vi "Quaternary_Layer2.vi"(2 "Debug Mode":bool, 3 "Elapsed Time (s)":dbl, 4 "State":enum16{"Edit", "Start", "Run", "End", "Idle"}(ring), 5 "Argument List In":string[](array[string])) -> (0 "Status Out":string, 1 "Argument List Out":string[](array[string]))   [LabVIEW 2011]
panel:
  in  "PH3 run":bool
  in  "AsH3 run":bool
  in  "In run":bool
  in  "Ga run":bool
  in  "PH3 Flow":dbl
  in  "AsH3 Flow":dbl
  in  "In Flow":dbl
  in  "Ga Flow":dbl
  in  "Cancel":bool
  in  "OK":bool
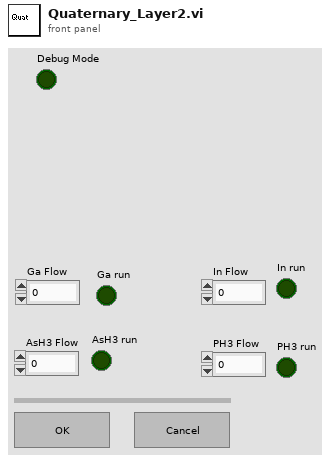
[diagram p1: front panel]
types:
  T1 = enum16{"Discrete", "Continuous", "Instantaneous"}
  T2 = enum32{"Invalid", "Default", "Floating", "Floating/Auto-Hide", "Modal"}
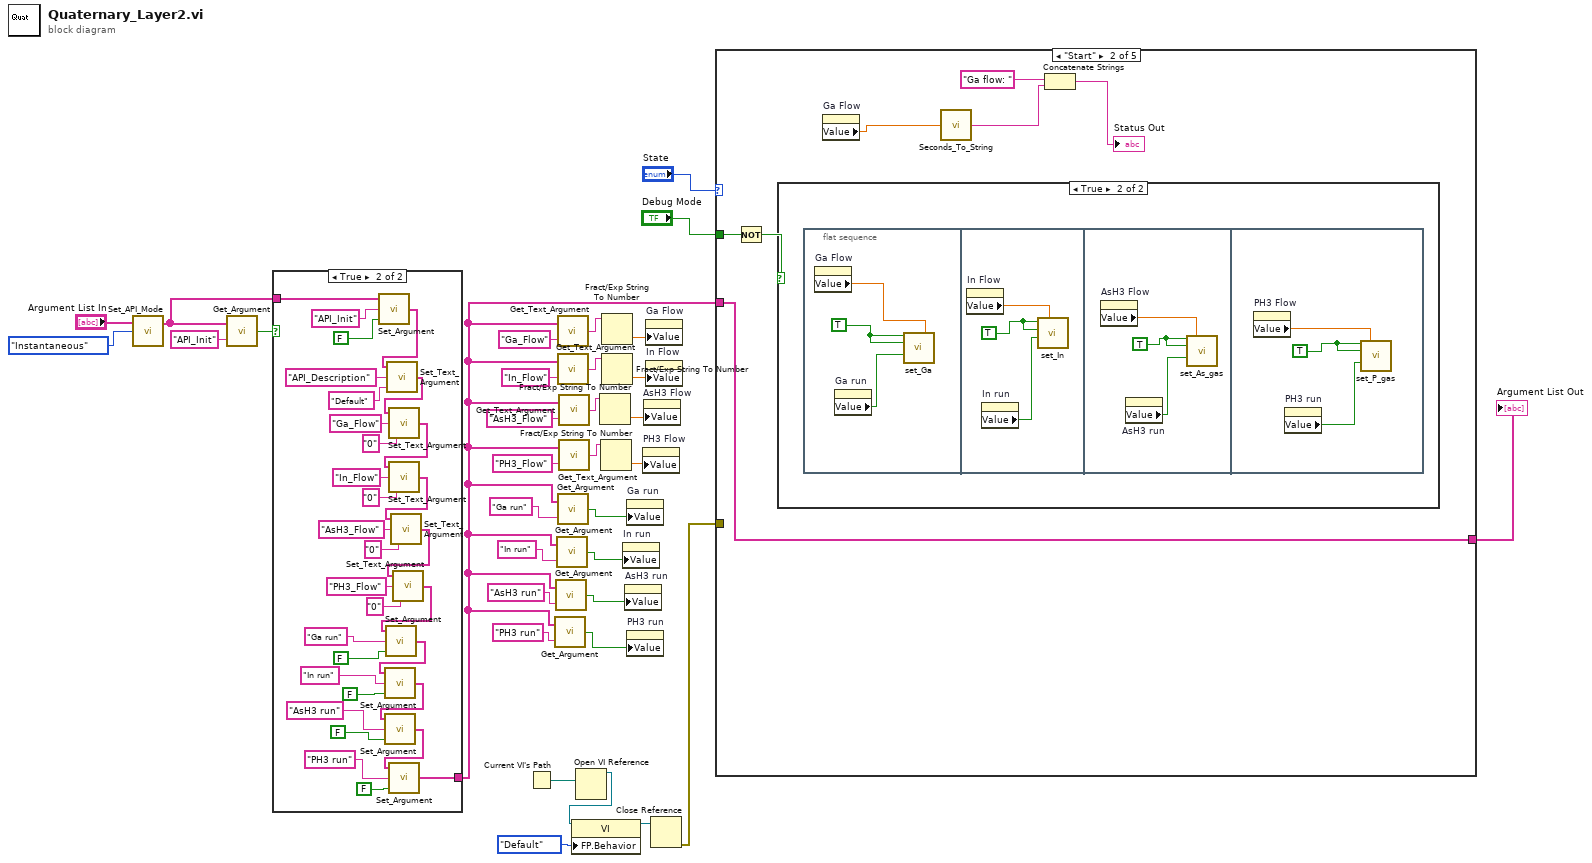
[diagram p0: block diagram]
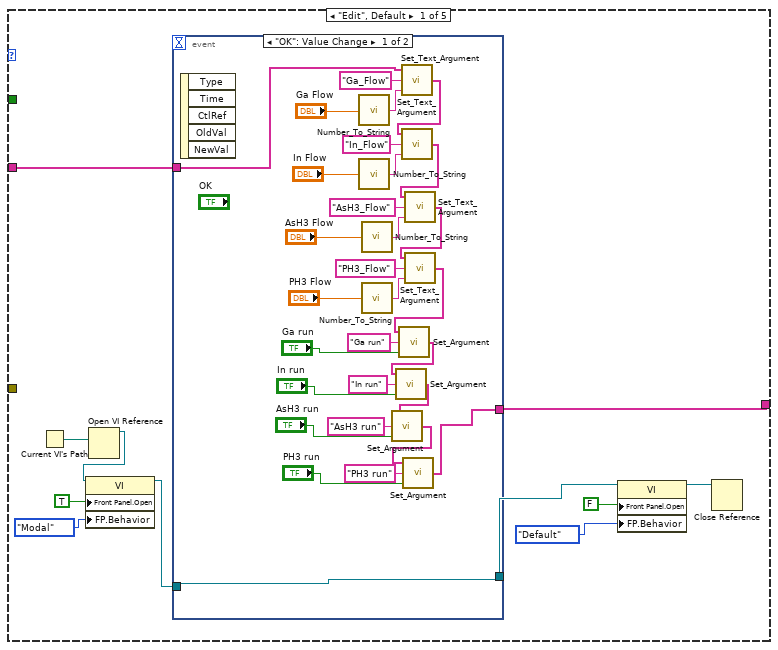
[diagram p3: hidden frame]
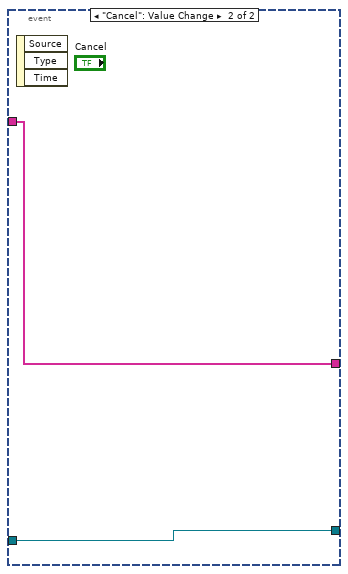
[diagram p4: hidden frame]
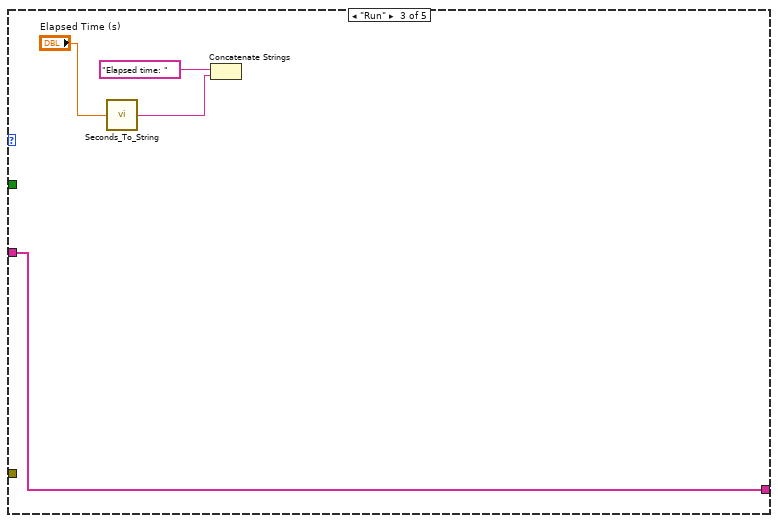
[diagram p6: hidden frame]
diagram:
  n1 = call "Set_API_Mode.vi"("API Mode"=T1."Instantaneous", "Argument List In"="Argument List In") -> ("Argument List Out"=w21:string[])  [unwired: 2 out]
  n2 = call "Get_Argument.vi"("Argument"="API_Init", "Argument List"=w21) -> ("Enabled"=w22:bool)
  n3 = case shown="True" w22 {
    tunnel: w21 -> [w35 w66]
    tunnel: [w35 w36] -> w1
    frame False {
    }
    frame True {
      n4 = call "Set_Argument.vi"("Enable"=FALSE, "Argument"="API_Init", "Argument List In"=w66) -> ("Argument List Out"=w63:string[])
      n5 = call "Set_Text_Argument.vi"("Text"="Default", "Argument"="API_Description", "Argument List In"=w63) -> ("Argument List Out"=w60:string[])
      n6 = call "Set_Text_Argument.vi"("Text"="0", "Argument"="Ga_Flow", "Argument List In"=w60) -> ("Argument List Out"=w55:string[])
      n7 = call "Set_Text_Argument.vi"("Text"="0", "Argument"="In_Flow", "Argument List In"=w55) -> ("Argument List Out"=w50:string[])
      n8 = call "Set_Text_Argument.vi"("Text"="0", "Argument"="AsH3_Flow", "Argument List In"=w50) -> ("Argument List Out"=w49:string[])
      n9 = call "Set_Text_Argument.vi"("Text"="0", "Argument"="PH3_Flow", "Argument List In"=w49) -> ("Argument List Out"=w40:string[])
      n10 = call "Set_Argument.vi"("Enable"=FALSE, "Argument"="Ga run", "Argument List In"=w40) -> ("Argument List Out"=w39:string[])
      n11 = call "Set_Argument.vi"("Enable"=FALSE, "Argument"="In run", "Argument List In"=w39) -> ("Argument List Out"=w38:string[])
      n12 = call "Set_Argument.vi"("Enable"=FALSE, "Argument"="AsH3 run", "Argument List In"=w38) -> ("Argument List Out"=w37:string[])
      n13 = call "Set_Argument.vi"("Enable"=FALSE, "Argument"="PH3 run", "Argument List In"=w37) -> ("Argument List Out"=w36:string[])
    }
  }
  n14 = Current VI's Path() -> (path=w30:path)
  n15 = call "Get_Argument.vi"("Argument"="PH3 run", "Argument List"=w1) -> ("Enabled"=w5:bool)
  n16 = call "Get_Argument.vi"("Argument"="AsH3 run", "Argument List"=w1) -> ("Enabled"=w6:bool)
  n17 = call "Get_Argument.vi"("Argument"="In run", "Argument List"=w1) -> ("Enabled"=w7:bool)
  n18 = call "Get_Text_Argument.vi"("Argument"="Ga_Flow", "Argument List"=w1) -> ("Text"=w17:string)
  n19 = call "Get_Text_Argument.vi"("Argument"="In_Flow", "Argument List"=w1) -> ("Text"=w15:string)
  n20 = call "Get_Argument.vi"("Argument"="Ga run", "Argument List"=w1) -> ("Enabled"=w8:bool)
  n21 = call "Get_Text_Argument.vi"("Argument"="AsH3_Flow", "Argument List"=w1) -> ("Text"=w13:string)
  n22 = call "Get_Text_Argument.vi"("Argument"="PH3_Flow", "Argument List"=w1) -> ("Text"=w11:string)
  n23 = Open VI Reference(vi path=w30) -> (vi reference=w29:refnum<vi>)  [unwired: 1 in, 5 out]
  n24 = property class="VI"(reference=w29, "FP.Behavior"=T2."Default" ("Front Panel Window:Behavior")) -> (reference out=w27:refnum<vi>)  [unwired: 1 in, 1 out]
  n25 = Fract/Exp String To Number(string=w13) -> (number=w12:dbl)  [unwired: 4 out]
  n26 = Fract/Exp String To Number(string=w11) -> (number=w10:dbl)  [unwired: 4 out]
  n27 = Fract/Exp String To Number(string=w17) -> (number=w16:dbl)  [unwired: 4 out]
  n28 = Fract/Exp String To Number(string=w15) -> (number=w14:dbl)  [unwired: 4 out]
  n29 = property on="In run" class="Bool (strict)"("Value"=w7) -> ()  [unwired: 2 in, 2 out]
  n30 = property on="AsH3 run" class="Bool (strict)"("Value"=w6) -> ()  [unwired: 2 in, 2 out]
  n31 = property on="Ga run" class="Bool (strict)"("Value"=w8) -> ()  [unwired: 2 in, 2 out]
  n32 = property on="PH3 run" class="Bool (strict)"("Value"=w5) -> ()  [unwired: 2 in, 2 out]
  n33 = property on="PH3 Flow" class="DigNum (strict)"("Value"=w10) -> ()  [unwired: 2 in, 2 out]
  n34 = property on="AsH3 Flow" class="DigNum (strict)"("Value"=w12) -> ()  [unwired: 2 in, 2 out]
  n35 = property on="Ga Flow" class="DigNum (strict)"("Value"=w16) -> ()  [unwired: 2 in, 2 out]
  n36 = property on="In Flow" class="DigNum (strict)"("Value"=w14) -> ()  [unwired: 2 in, 2 out]
  n37 = Close Reference(reference=w27) -> (error out=w26:errorcluster)  [unwired: 1 in]
  n38 = case shown="\"Start\"" "State" {
    tunnel: [w77 w116 w129 w133 w134] -> w33
    tunnel: w1 -> [w76 w116 w129 w133 w134]
    tunnel: "Debug Mode" -> [_ w115 _ _ _]
    tunnel: w26 -> [_ _ _ _ _]
    frame "Edit", Default {
      n39 = Current VI's Path() -> (path=w71:path)
      n40 = Open VI Reference(vi path=w71) -> (vi reference=w70:refnum<vi>)  [unwired: 1 in, 5 out]
      n41 = property class="VI"(reference=w70, "Front Panel.Open"=TRUE ("Front Panel Window:Open"), "FP.Behavior"=T2."Modal" ("Front Panel Window:Behavior")) -> (reference out=w74:refnum<vi>)  [unwired: 1 in, 1 out]
      n42 = event shown="[0] \"OK\": Value Change" {
        selector: _ -> [_ _]
        dyn-events: _ -> [_ _]
        timeout: _ -> [_ _]
        tunnel: w76 -> [w104 w108]
        tunnel: [w78 w108] -> w77
        tunnel: [w107 w109] -> w73
        tunnel: w74 -> [w107 w109]
        event "OK": Value Change {
          n43 = event-data() -> ()  [unwired: 6 out]
          n44 = call "Number_To_String.vi"("Number"="Ga Flow") -> ("String"=w105:string)
          n45 = call "Number_To_String.vi"("Number"="In Flow") -> ("String"=w101:string)
          n46 = call "Number_To_String.vi"("Number"="AsH3 Flow") -> ("String"=w97:string)
          n47 = call "Number_To_String.vi"("Number"="PH3 Flow") -> ("String"=w93:string)
          n48 = call "Set_Text_Argument.vi"("Text"=w105, "Argument"="Ga_Flow", "Argument List In"=w104) -> ("Argument List Out"=w100:string[])
          n49 = call "Set_Text_Argument.vi"("Text"=w101, "Argument"="In_Flow", "Argument List In"=w100) -> ("Argument List Out"=w96:string[])
          n50 = call "Set_Text_Argument.vi"("Text"=w97, "Argument"="AsH3_Flow", "Argument List In"=w96) -> ("Argument List Out"=w92:string[])
          n51 = call "Set_Text_Argument.vi"("Text"=w93, "Argument"="PH3_Flow", "Argument List In"=w92) -> ("Argument List Out"=w82:string[])
          n52 = call "Set_Argument.vi"("Enable"="Ga run", "Argument"="Ga run", "Argument List In"=w82) -> ("Argument List Out"=w81:string[])
          n53 = call "Set_Argument.vi"("Enable"="In run", "Argument"="In run", "Argument List In"=w81) -> ("Argument List Out"=w80:string[])
          n54 = call "Set_Argument.vi"("Enable"="AsH3 run", "Argument"="AsH3 run", "Argument List In"=w80) -> ("Argument List Out"=w79:string[])
          n55 = call "Set_Argument.vi"("Enable"="PH3 run", "Argument"="PH3 run", "Argument List In"=w79) -> ("Argument List Out"=w78:string[])
        }
        event "Cancel": Value Change {
          n56 = event-data() -> ()  [unwired: 4 out]
        }
      }
      n57 = property class="VI"(reference=w73, "Front Panel.Open"=FALSE ("Front Panel Window:Open"), "FP.Behavior"=T2."Default" ("Front Panel Window:Behavior")) -> (reference out=w67:refnum<vi>)  [unwired: 1 in, 1 out]
      n58 = Close Reference(reference=w67) -> ()  [unwired: 1 in, 1 out]
    }
    frame "Start" {
      n59 = Not(x=w115) -> (.not. x?=w114:bool)
      n60 = case shown="True" w114 {
        frame False {
        }
        frame True {
          n61 = flat-sequence {
            frame #0 {
              w119 = TRUE ("Ga Active")
              n62 = property on="Ga Flow" class="DigNum (strict)"() -> ("Value"=w118:dbl)  [unwired: 2 in, 2 out]
              n63 = property on="Ga run" class="Bool (strict)"() -> ("Value"=w117:bool)  [unwired: 2 in, 2 out]
              n64 = call "set_Ga.vi"("Ga Active"=w119, "Ga Flow 1"=w118, "Ga Bubbler"=w119, "Ga Run"=w117) -> ()  [unwired: 4 in, 8 out]
            }
            frame #1 {
              w122 = TRUE ("Ga Active")
              n65 = property on="In Flow" class="DigNum (strict)"() -> ("Value"=w121:dbl)  [unwired: 2 in, 2 out]
              n66 = property on="In run" class="Bool (strict)"() -> ("Value"=w120:bool)  [unwired: 2 in, 2 out]
              n67 = call "set_In.vi"("Indium Flow"=w121, "In Run"=w120, "In Bubbler"=w122, "In Active"=w122) -> ()  [unwired: 1 in, 5 out]
            }
            frame #2 {
              w124 = TRUE ("Ga Active")
              n68 = property on="AsH3 Flow" class="DigNum (strict)"() -> ("Value"=w125:dbl)  [unwired: 2 in, 2 out]
              n69 = property on="AsH3 run" class="Bool (strict)"() -> ("Value"=w123:bool)  [unwired: 2 in, 2 out]
              n70 = call "set_As_gas.vi"("As_Gas Active"=w124, "As_Gas Flow"=w125, "As_Gas In"=w124, "As_Gas Run"=w123) -> ()  [unwired: 2 in, 10 out]
            }
            frame #3 {
              w128 = TRUE ("Ga Active")
              n71 = property on="PH3 Flow" class="DigNum (strict)"() -> ("Value"=w127:dbl)  [unwired: 2 in, 2 out]
              n72 = property on="PH3 run" class="Bool (strict)"() -> ("Value"=w126:bool)  [unwired: 2 in, 2 out]
              n73 = call "set_P_gas.vi"("P_Gas Active"=w128, "P_Gas Flow"=w127, "P_Gas In"=w128, "P_Gas Run"=w126) -> ()  [unwired: 2 in, 10 out]
            }
          }
        }
      }
      n74 = property on="Ga Flow" class="DigNum (strict)"() -> ("Value"=w111:dbl)  [unwired: 2 in, 2 out]
      n75 = call "Seconds_To_String.vi"("Seconds"=w111) -> ("Output String"=w112:string)
      n76 = Concatenate Strings("Ga flow: " ("string"), w112) -> (→"Status Out":string)
    }
    frame "Run" {
      n77 = call "Seconds_To_String.vi"("Seconds"="Elapsed Time (s)") -> ("Output String"=w130:string)
      n78 = Concatenate Strings("Elapsed time: " ("string"), w130) -> ()  [unwired: 1 out]
    }
    frame "End" {
    }
    frame "Idle" {
    }
  }
  "Argument List Out" <- w33
